vi "variable on-off blinker.vi"() -> ()   [LabVIEW 2018]
panel:
  in  "Boolean 2":bool
  in  "Off Time":dbl
  in  "On Time":dbl
  out "Boolean":bool
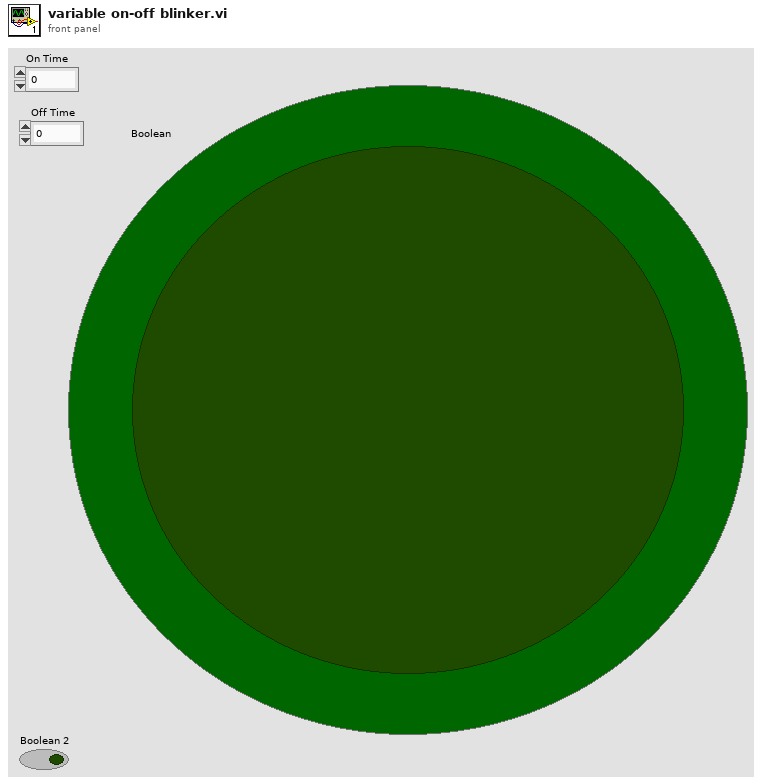
[diagram p1: front panel]
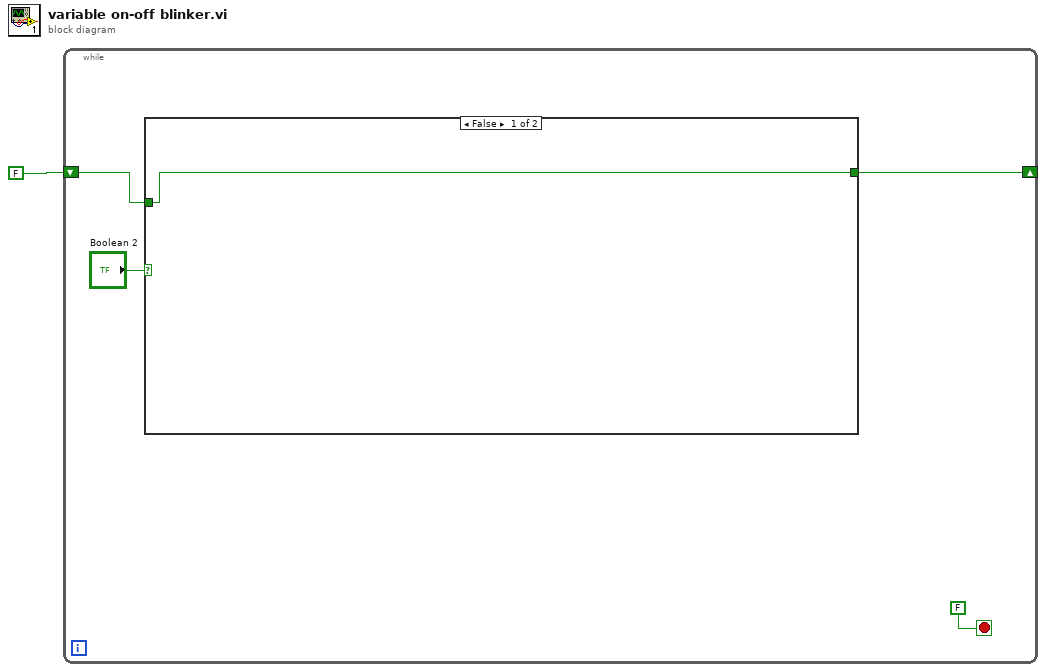
[diagram p0: block diagram]
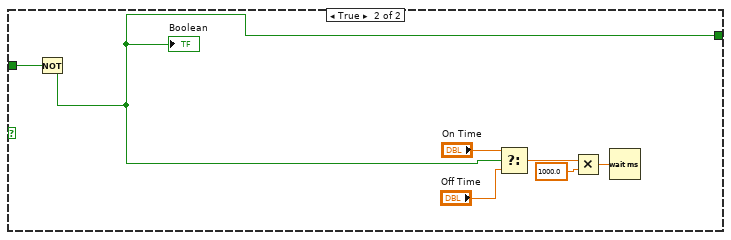
[diagram p2: hidden frame]
diagram:
  n1 = while {
    shift-right: [w3] -> _
    shift-left: FALSE -> [w4]
    stop <- FALSE stop-if-true
    n2 = case shown="False" "Boolean 2" {
      tunnel: w4 -> [w6 w13]
      tunnel: [w6 w9] -> w3
      frame False {
      }
      frame True {
        n3 = Not(x=w13) -> (.not. x?=w9:bool)
        "Boolean" <- w9
        n4 = Select(t="On Time", s=w9, f="Off Time") -> (s? t:f=w12:dbl)
        n5 = Multiply(x=w12, y=1000.0) -> (x*y=w7:dbl)
        n6 = Wait (ms)(milliseconds to wait=w7) -> ()  [unwired: 1 out]
      }
    }
  }
